vi "PXI-Refresh AO Buffer (queue).vi"(6 "BufferSize":i32, 8 "error in (no error)":errorcluster, 9 "AO Waveforms In":dbl[][](array[numeric]), 10 "AO Tasks":T1[](array[typedef]), 11 "Wait for buffer space? (T)":bool=TRUE) -> (0 "error out (no error)":errorcluster, 3 "AO Waveforms Out":dbl[][](array[numeric]))   [LabVIEW 2020]
uses:
  Type Defs/Task Struct.ctl
  PXI Globals.vi
panel:
  out "Waveform Graph":dbl[][](graph)
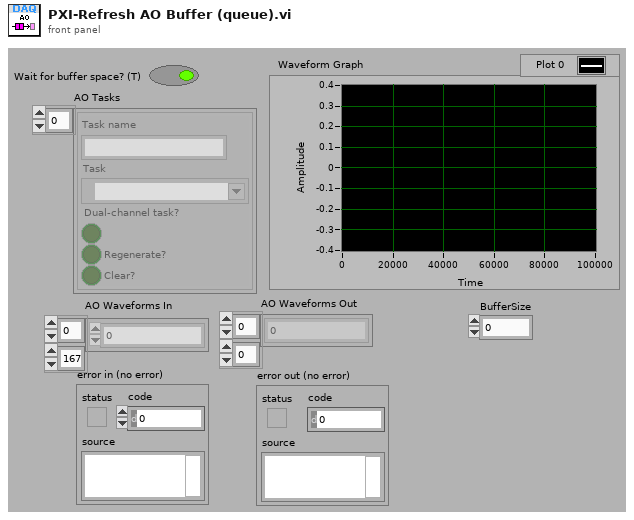
[diagram p1: front panel]
types:
  T1 = typedef "Task Struct.ctl" = cluster{"Task name":string, "Task":refnum<k21>, "Dual-channel task?":bool, "Regenerate?":bool, "Clear?":bool}
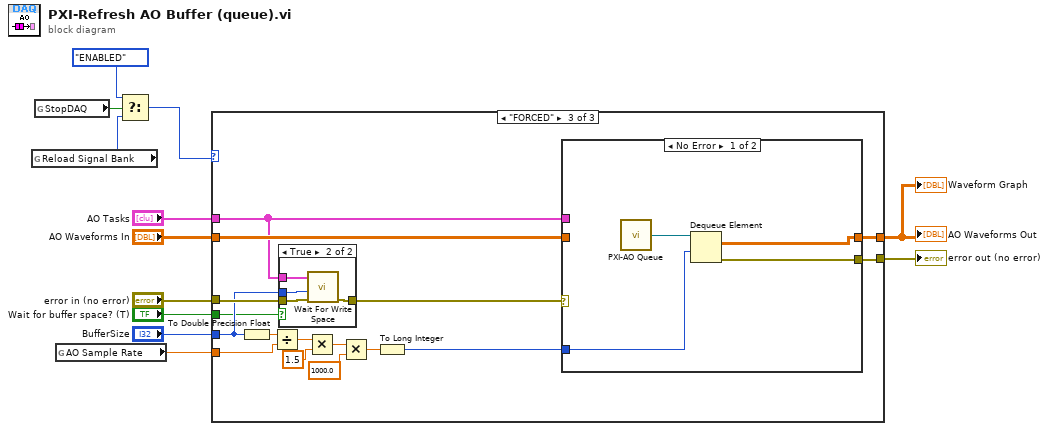
[diagram p0: block diagram]
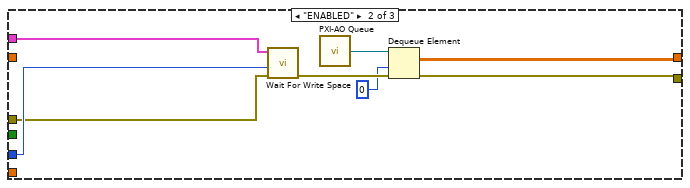
[diagram p3: hidden frame]
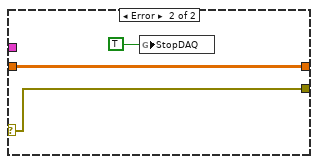
[diagram p5: hidden frame]
diagram:
  n1 = global read "PXI Globals.vi" "Reload Signal Bank"() -> (w7:enum32{"OFF", "ENABLED", "FORCED"})
  n2 = global read "PXI Globals.vi" "StopDAQ"() -> (w4:bool)
  n3 = global read "PXI Globals.vi" "AO Sample Rate"() -> (w2:dbl)
  n4 = Select(t=enum16{"OFF", "ENABLED", "FORCED"}."ENABLED", s=w4, f=w7) -> (s? t:f=w6:enum32{"OFF", "ENABLED", "FORCED"})
  n5 = case shown="\"FORCED\"" w6 {
    tunnel: "error in (no error)" -> [w14 w20 w38]
    tunnel: [w14 w17 w37] -> w11
    tunnel: "AO Waveforms In" -> [w13 _ w35]
    tunnel: [w13 w16 w36] -> w5
    tunnel: "AO Tasks" -> [_ w22 w25]
    tunnel: "BufferSize" -> [_ w21 w28]
    tunnel: w2 -> [_ _ w27]
    tunnel: "Wait for buffer space? (T)" -> [_ _ w26]
    frame "OFF", Default {
    }
    frame "ENABLED" {
      n6 = call "Wait For Write Space.vi"("error in (no error)"=w20, "BufferSize"=w21, "AO Tasks"=w22) -> ("error out"=w18:errorcluster)  [unwired: 6 in, 2 out]
      n7 = call "PXI-AO Queue.vi"() -> ("Queue"=w19:refnum<queue>)  [unwired: 15 in]
      n8 = Dequeue Element(queue=w19, timeout in ms (-1)=0, error in (no error)=w18) -> (element=w16:dbl[][], error out=w17:errorcluster)  [unwired: 2 out]
    }
    frame "FORCED" {
      n9 = To Double Precision Float(number=w28) -> (double precision float=w29:dbl)
      n10 = Divide(x=w29, y=w27) -> (x/y=w30:dbl)
      n11 = case shown="True" w26 {
        tunnel: w38 -> [w39 w43]
        tunnel: w28 -> [_ w42]
        tunnel: w25 -> [_ w41]
        tunnel: [w39 w40] -> w24
        frame False {
        }
        frame True {
          n12 = call "Wait For Write Space.vi"("error in (no error)"=w43, "BufferSize"=w42, "AO Tasks"=w41) -> ("error out"=w40:errorcluster)  [unwired: 6 in, 2 out]
        }
      }
      n13 = Multiply(x=w30, y=1.5) -> (x*y=w32:dbl)
      n14 = Multiply(x=w32, y=1000.0) -> (x*y=w34:dbl)
      n15 = To Long Integer(number=w34) -> (32bit integer=w23:i32)
      n16 = case shown="No Error" w24 {
        selector: w24 -> [_ w48]
        tunnel: [w46 w48] -> w37
        tunnel: [w45 w50] -> w36
        tunnel: w35 -> [_ w50]
        tunnel: w25 -> [_ _]
        tunnel: w23 -> [w44 _]
        frame No Error {
          n17 = call "PXI-AO Queue.vi"() -> ("Queue"=w47:refnum<queue>)  [unwired: 15 in]
          n18 = Dequeue Element(queue=w47, timeout in ms (-1)=w44) -> (element=w45:dbl[][], error out=w46:errorcluster)  [unwired: 1 in, 2 out]
        }
        frame Error {
          n19 = global write "PXI Globals.vi" "StopDAQ"(TRUE) -> ()
        }
      }
    }
  }
  "AO Waveforms Out" <- w5
  "error out (no error)" <- w11
  "Waveform Graph" <- w5
